vi "Add Modules to Slot List (Timing).vi"(8 "error in (no error)":errorcluster, 9 "TimingGrp in":refnum<class "TimingGrp.lvclass">, 11 "SlotMod List":string[](array[string])) -> (0 "error out":errorcluster, 3 "Slot Mod Lilst":string[](array[string]))   [LabVIEW 2012, in "Configuration Grandmaster.lvlib" / "TimingGrp.lvclass"]
uses:
  TimingGrp.lvclass
  TimingGrp.lvclass/TimingGrp.ctl
  Class Chan Group/ChanGrp.lvclass
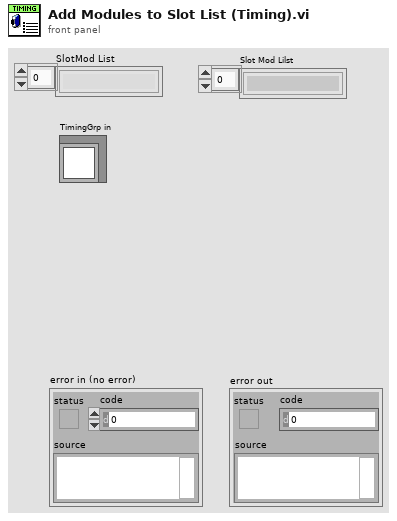
[diagram p1: front panel]
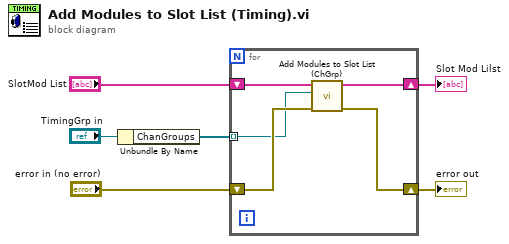
[diagram p0: block diagram]
diagram:
  n1 = Unbundle By Name("TimingGrp in") -> ("ChanGroups"=w3:refnum<class "ChanGrp.lvclass">[])
  n2 = for {
    shift-right: [w10] -> w2
    shift-left: "SlotMod List" -> [w11]
    shift-right: [w8] -> w4
    shift-left: "error in (no error)" -> [w9]
    tunnel: w3 -> [w7] mode=indexing
    n3 = call "Add Modules to Slot List (ChGrp).vi"("error in (no error)"=w9, "ChanGrp.lvclass"=w7, "SlotMod List in"=w11) -> ("error out"=w8:errorcluster, "SlotMod List out"=w10:string[])  [unwired: 7 in]
  }
  "Slot Mod Lilst" <- w2
  "error out" <- w4
